vi "Test_AbstractTransport_Write_Error.vi"(8 "error in (no error)":errorcluster, 11 "TestCase in":refnum<class "TestITransport.lvclass">) -> (0 "error out":errorcluster, 3 "TestCase out":refnum<class "TestITransport.lvclass">)   [LabVIEW 2017, in "TestITransport.lvclass"]
uses:
  TestITransport.lvclass
  Source/ITransport/ITransport.lvclass
panel:
  out "Return Error":errorcluster
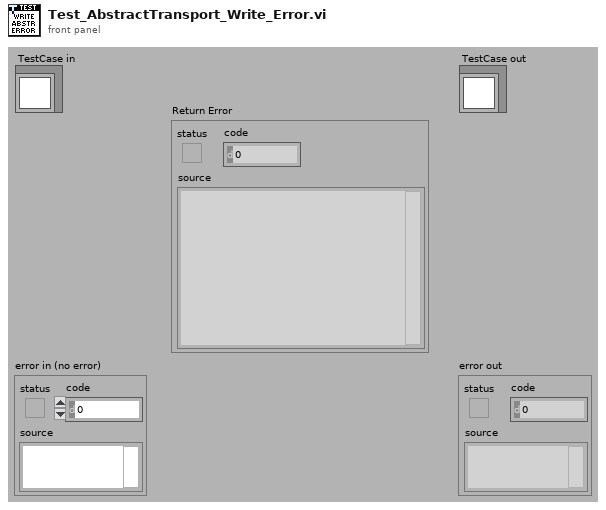
[diagram p1: front panel]
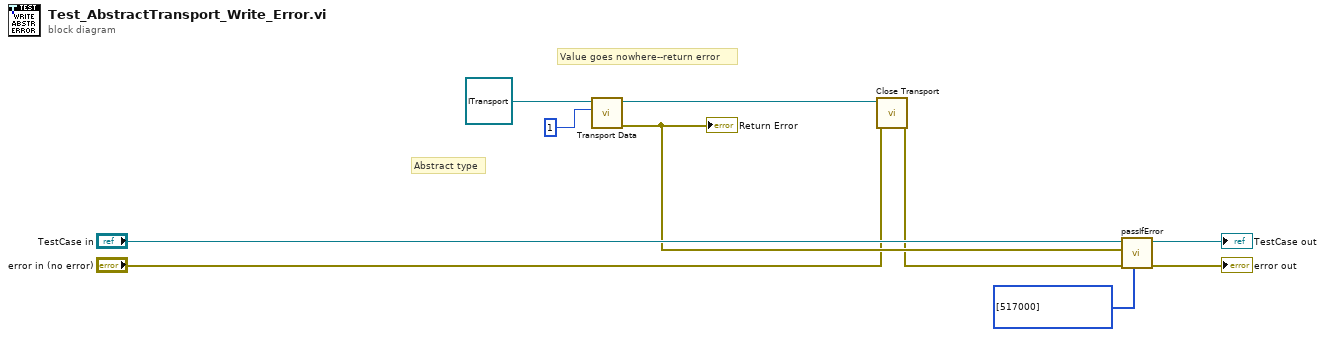
[diagram p0: block diagram]
diagram:
  # "Value goes nowhere--return error"
  # "Abstract type"
  n1 = call "Transport Data.vi"("Value"=1, "ITransport in"=refnum<class "ITransport.lvclass"> refnum ("ITransport.lvclass")) -> ("error out"=w4:errorcluster, "ITransport out"=w3:refnum<class "ITransport.lvclass">)  [unwired: 8 in]
  "Return Error" <- w4
  n2 = call-dynamic "Close Transport.vi"("error in (no error)"="error in (no error)", "ITransport in"=w3) -> ("error out"=w1:errorcluster)  [unwired: 9 in]
  n3 = call-dynamic "passIfError.vi"("passing error codes (default = any error code)"=i32[] [517000], "error in (no error)"=w1, "error"=w4, "TestCase in"="TestCase in") -> ("error out"=→"error out":errorcluster, "TestCase out"=→"TestCase out":refnum<class "TestITransport.lvclass">)  [unwired: 6 in]
